vi "POV to Buttons.vi"(11 "POV Input":dbl) -> (0 "Right":bool, 1 "Down":bool, 2 "Left":bool, 3 "Up":bool)   [LabVIEW 2014]
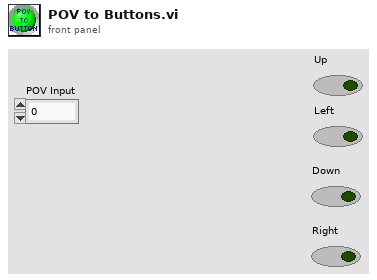
[diagram p1: front panel]
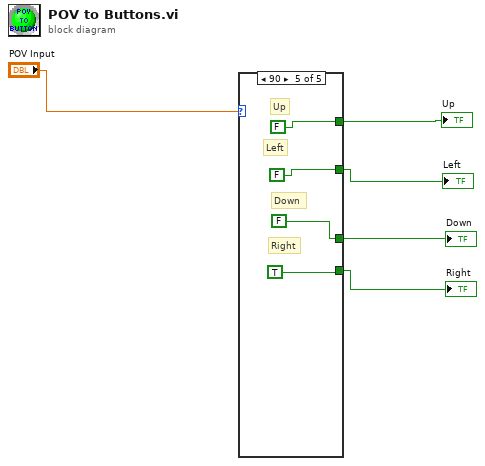
[diagram p0: block diagram]
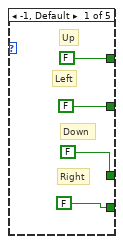
[diagram p2: hidden frame]
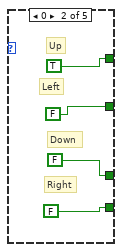
[diagram p3: hidden frame]
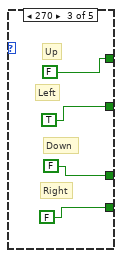
[diagram p4: hidden frame]
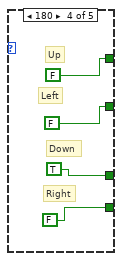
[diagram p5: hidden frame]
diagram:
  n1 = case shown="90" "POV Input" {
    tunnel: [FALSE TRUE FALSE FALSE FALSE] -> w4
    tunnel: [FALSE FALSE TRUE FALSE FALSE] -> w3
    tunnel: [FALSE FALSE FALSE FALSE TRUE] -> w1
    tunnel: [FALSE FALSE FALSE TRUE FALSE] -> w2
    frame -1, Default {
      # "Right"
      # "Down"
      # "Left"
      # "Up"
    }
    frame 0 {
      # "Right"
      # "Down"
      # "Left"
      # "Up"
    }
    frame 270 {
      # "Right"
      # "Down"
      # "Left"
      # "Up"
    }
    frame 180 {
      # "Right"
      # "Down"
      # "Left"
      # "Up"
    }
    frame 90 {
      # "Right"
      # "Down"
      # "Left"
      # "Up"
    }
  }
  "Up" <- w4
  "Left" <- w3
  "Down" <- w2
  "Right" <- w1
